vi "CRYPEAQ HannWin.vi"(11 "NF":dbl) -> (3 "hw":dbl[](array[numeric]))   [LabVIEW 2013]
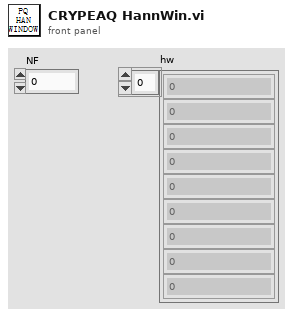
[diagram p1: front panel]
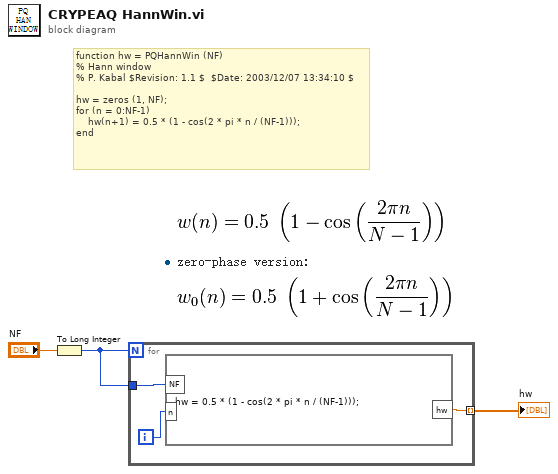
[diagram p0: block diagram]
diagram:
  # "function hw = PQHannWin (NF)\n% Hann window\n% P. Kabal $Revision: 1.1 $  $Date: 2003/12/07 13:34:10 $\n\nhw = zeros (1, NF);\nfor (n = 0:NF-1)\n    hw(n+1) = 0.5 * (1 - cos(2 * pi * n / (NF-1)));\nend"
  n1 = To Long Integer(number="NF") -> (32bit integer=w3:i32)
  n2 = for {
    N: w3 -> [_]
    tunnel: [w6] -> w2 mode=indexing
    tunnel: w3 -> [w4]
    i -> [w5]
    n3 = formula code="hw = 0.5 * (1 - cos(2 * pi * n / (NF-1)));"("n"=w5, "NF"=w4) -> ("hw"=w6:dbl)
  }
  "hw" <- w2
